vi "Stop Core.vi"(10 "final error code":i32, 11 "RootModel in":refnum<class "RootModel.lvclass">) -> (3 "RootModel out":refnum<class "RootModel.lvclass">)   [LabVIEW 2019, in "RootModel.lvlib" / "RootModel.lvclass"]
uses:
  <vilib>/gpm_packages/@cs/mva-core/Source/RootModel/RootModel/RootModel.lvclass
  C:/Program Files/National Instruments/LabVIEW 2019/vi.lib/gpm_packages/@cs/mva-core/Source/IObserver/IObserver/IObserver.lvclass
  <vilib>/gpm_packages/@cs/mva-core/Source/RootModel/RootModel/RootModel.lvclass/RootModel.ctl
  <vilib>/gpm_packages/@cs/mva-core/Source/IObserver/IObserver/IObserver.lvclass/IObserver.ctl
  <vilib>/gpm_packages/@cs/event-logger/Source/Composed Log/LoggerReference/Close Local Event Log.vi
  <vilib>/gpm_packages/@cs/mva-core/Source/IModel/IModel/IModel.lvclass
  <vilib>/gpm_packages/@cs/mva-core/Source/IObserver/IObserver/IObserver.lvclass
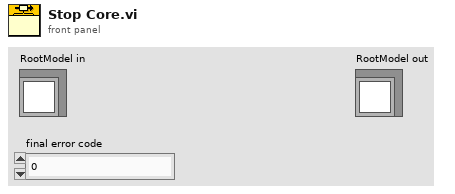
[diagram p1: front panel]
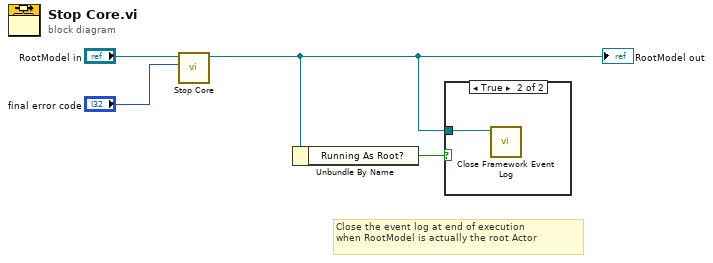
[diagram p0: block diagram]
diagram:
  # "Close the event log at end of execution\nwhen RootModel is actually the root Actor"
  n1 = call-parent "Stop Core.vi"("final error code"="final error code", "IObserver in"="RootModel in") -> ("IObserver out"=w2:refnum<class "RootModel.lvclass">)  [unwired: 9 in]
  "RootModel out" <- w2
  n2 = Unbundle By Name(w2) -> ("Running As Root?"=w1:bool)
  n3 = case shown="True" w1 {
    tunnel: w2 -> [_ w5]
    frame False {
    }
    frame True {
      n4 = call <vilib>:"Close Framework Event Log.vi"("IObserver in"=w5) -> ()  [unwired: 11 in]
    }
  }
